vi "Read.vi"(11 "Variant in":refnum<class "Variant.lvclass">) -> (2 "Value":variant)   [LabVIEW 2020, in "Promises.lvlib" / "Variant.lvclass"]
uses:
  Variant.lvclass
  Variant.lvclass/Variant.ctl
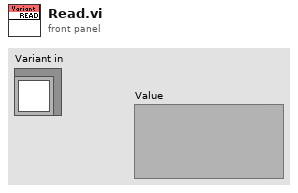
[diagram p1: front panel]
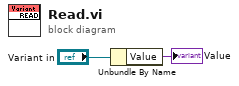
[diagram p0: block diagram]
diagram:
  n1 = Unbundle By Name("Variant in") -> ("Value"=→"Value":variant)
